vi "HexapodInitializeHardware.vi"(8 "error in (no error)":errorcluster, 11 "HexapodPI in":refnum<class "HexapodPI.lvclass">) -> (0 "error out":errorcluster, 2 "devaddress":string, 3 "HexapodPI out":refnum<class "HexapodPI.lvclass">)   [LabVIEW 2020, in "HexapodPI.lvclass"]
uses:
  HexapodPI.lvclass
  HexapodPI.lvclass/HexapodPI.ctl
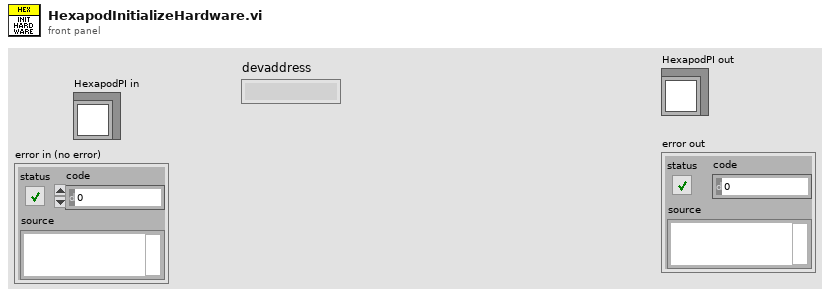
[diagram p1: front panel]
types:
  T1 = cluster{"connection ID":refnum<k5>, "VISA resource name out":refnum<visa-resource-name>, "connectiontype":enum16{"TCPIP", "Serial"}}
  T2 = cluster{"connection ID":refnum<k5>, "VISA resource name":refnum<visa-resource-name>, "Selector":enum16{"TCPIP", "Serial"}}
  T3 = cluster{"connection ID":refnum<k5>, "VISA Refnum out":refnum<visa-resource-name>, "Selector":enum16{"TCPIP", "Serial"}}
  T4 = cluster{"Strut 1 motion error":bool, "Strut 2 motion error":bool, "Strut 3 motion error":bool, "Strut 4 motion error":bool, "Strut 5 motion error":bool, "Strut 6 motion error":bool, "Axis A motion error":bool, "Axis B motion error":bool, "Strut 1 in motion":bool, "Strut 2 in motion":bool, "Strut 3 in motion":bool, "Strut 4 in motion":bool, "Strut 5 in motion":bool, "Strut 6 in motion":bool, "Axis A in motion":bool, "Axis B in motion":bool, "Hexapod is Initialized":bool, "Stage A is Initialized":bool, "Stage B is Initialized":bool, "Initialisation in progress":bool}
  T5 = typedef "PivotPoint_TypDef.ctl" = cluster{"R":cluster{"Value":dbl, "Min":dbl, "Max":dbl, "StepSize":dbl, "Tolerance":dbl, "ValueActual":dbl}, "S":cluster{"Value":dbl, "Min":dbl, "Max":dbl, "StepSize":dbl, "Tolerance":dbl, "ValueActual":dbl}, "T":cluster{"Value":dbl, "Min":dbl, "Max":dbl, "StepSize":dbl, "Tolerance":dbl, "ValueActual":dbl}}
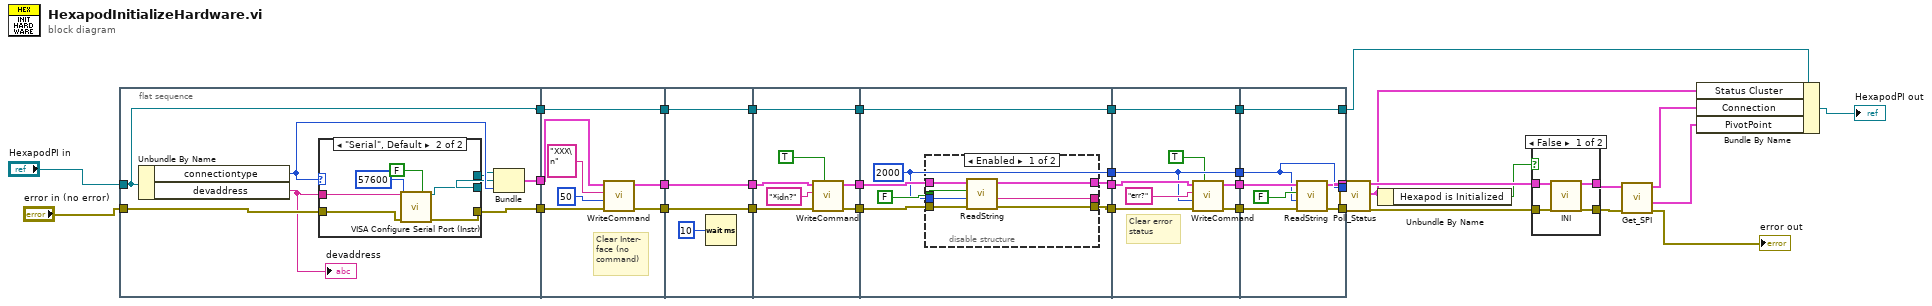
[diagram p0: block diagram]
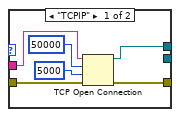
[diagram p3: hidden frame]
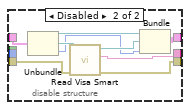
[diagram p4: hidden frame]
diagram:
  n1 = flat-sequence {
    tunnel: "error in (no error)" -> [w44]
    tunnel: [w43] -> w36
    tunnel: [w40] -> w35
    tunnel: "HexapodPI in" -> [w37]
    tunnel: [w37] -> w11
    tunnel: [w62] -> w34
    tunnel: [w60] -> w33
    tunnel: w36 -> [w61]
    tunnel: w35 -> [w58]
    tunnel: w11 -> [w57]
    tunnel: [w57] -> w8
    tunnel: w34 -> [w66]
    tunnel: [w66] -> w32
    tunnel: [w65] -> w31
    tunnel: w33 -> [w65]
    tunnel: [w64] -> w9
    tunnel: w8 -> [w64]
    tunnel: w32 -> [w74]
    tunnel: [w69] -> w30
    tunnel: w31 -> [w72]
    tunnel: [w71] -> w29
    tunnel: [w68] -> w10
    tunnel: w9 -> [w68]
    tunnel: w30 -> [w81]
    tunnel: [w76] -> w28
    tunnel: w29 -> [w79]
    tunnel: [w78] -> w27
    tunnel: [w77] -> w26
    tunnel: w10 -> [w75]
    tunnel: [w75] -> w6
    tunnel: w28 -> [w105]
    tunnel: [w104] -> w25
    tunnel: w27 -> [w101]
    tunnel: [w102] -> w24
    tunnel: w26 -> [w100]
    tunnel: [w100] -> w23
    tunnel: [w98] -> w7
    tunnel: w6 -> [w98]
    tunnel: w25 -> [w112]
    tunnel: [w111] -> w15
    tunnel: w24 -> [w109]
    tunnel: [w108] -> w14
    tunnel: w23 -> [w107]
    tunnel: [w107] -> w19
    tunnel: [w106] -> w5
    tunnel: w7 -> [w106]
    frame #0 {
      n2 = Unbundle By Name(w37) -> ("connectiontype"=w41:enum16{"TCPIP", "Serial"}, "devaddress"=w42:string)
      "devaddress" <- w42
      n3 = case shown="\"Serial\", Default" w41 {
        tunnel: w44 -> [w48 w52]
        tunnel: [w47 w55] -> w43
        tunnel: [w46 _] -> w38
        tunnel: w42 -> [w45 w53]
        tunnel: [_ w56] -> w39
        frame "TCPIP" {
          n4 = TCP Open Connection(address=w45, remote port or service name=u16 50000, timeout ms (60000)=5000, error in (no error)=w48) -> (connection ID=w46:refnum<k5>, error out=w47:errorcluster)  [unwired: 1 in]
        }
        frame "Serial", Default {
          n5 = call "VISA Configure Serial Port (Instr).vi"("VISA resource name"=w53, "Enable Termination\nChar (T)"=FALSE ("Enable Termination\nChar (T)"), "baud rate (9600)"=u32 57600, "error in (no error)"=w52) -> ("VISA resource name out"=w56:refnum<visa-resource-name>, "error out"=w55:errorcluster)  [unwired: 10 in]
        }
      }
      n6 = Bundle("connection ID"=w38, "VISA resource name out"=w39, "connectiontype"=w41) -> (w40:T1)  [unwired: 1 in]
    }
    frame #1 {
      # "Clear Inter-\nface (no\ncommand)"
      n7 = call "WriteCommand.vi"("error in (no error)"=w61, "timeout ms (0)"=50, "String"="XXX\n" ("Interface clear"), "Connection"=w58) -> ("error out"=w62:errorcluster, "Connection out"=w60:T2)  [unwired: 6 in]
    }
    frame #2 {
      n8 = Wait (ms)(milliseconds to wait=u32 10) -> ()  [unwired: 1 out]
    }
    frame #3 {
      n9 = call "WriteCommand.vi"("Attach Linefeed"=TRUE, "error in (no error)"=w74, "String"="*idn?" ("String to Send"), "Connection"=w72) -> ("error out"=w69:errorcluster, "Connection out"=w71:T2)  [unwired: 6 in]
    }
    frame #4 {
      w77 = 2000 ("timeout ms (0)")
      n10 = disable-structure shown="Enabled" {
        disable-tunnel: w81 -> [w88 w96]
        disable-tunnel: [w87 w89] -> _
        disable-tunnel: FALSE ("Strip spaces?") -> [w86 _]
        disable-tunnel: w79 -> [w85 w95]
        disable-tunnel: [w84 w92] -> w78
        disable-tunnel: w77 -> [w83 _]
        disable-tunnel: [w82 w97] -> w76
        frame Enabled {
          n11 = call "ReadString.vi"("error in (no error)"=w88, "timeout ms (0)"=w83, "Trim Spaces"=w86, "Connection"=w85) -> ("error out"=w82:errorcluster, "String out"=w87:string, "Connection out"=w84:T2)  [unwired: 5 in]
        }
        frame Disabled {
          n12 = Unbundle(w95) -> ("connection ID"=w93:refnum<k5>, "VISA resource name"=w94:refnum<visa-resource-name>, "Selector"=w90:enum16{"TCPIP", "Serial"})
          n13 = call "Read Visa Smart.vi"("error in (no error)"=w96, "VISA Refnum in"=w94) -> ("error out"=w97:errorcluster, "String"=w89:string, "VISA Refnum out"=w91:refnum<visa-resource-name>)  [unwired: 7 in]
          n14 = Bundle("connection ID"=w93, "VISA Refnum out"=w91, "Selector"=w90) -> (w92:T3)  [unwired: 1 in]
        }
      }
    }
    frame #5 {
      # "Clear error\nstatus"
      n15 = call "WriteCommand.vi"("Attach Linefeed"=TRUE, "error in (no error)"=w105, "timeout ms (0)"=w100, "String"="err?" ("String to Send"), "Connection"=w101) -> ("error out"=w104:errorcluster, "Connection out"=w102:T2)  [unwired: 5 in]
    }
    frame #6 {
      n16 = call "ReadString.vi"("error in (no error)"=w112, "timeout ms (0)"=w107, "Trim Spaces"=FALSE ("Strip spaces?"), "Connection"=w109) -> ("error out"=w111:errorcluster, "Connection out"=w108:T2)  [unwired: 5 in, 1 out]
    }
  }
  n17 = call "Poll_Status.vi"("Connection"=w14, "timeout ms (0)"=w19, "error in"=w15) -> ("Connection out"=w17:T2, "Status Cluster"=w4:T4, "error out"=w18:errorcluster)  [unwired: 14 in]
  n18 = Unbundle By Name(w4) -> ("Hexapod is Initialized"=w16:bool)
  n19 = case shown="False" w16 {
    tunnel: w17 -> [w116 w118]
    tunnel: [w115 w118] -> w20
    tunnel: w18 -> [w114 w117]
    tunnel: [w113 w117] -> w21
    frame False {
      n20 = call "INI.vi"("Connection"=w116, "error in"=w114) -> ("Connection out"=w115:T2, "error out"=w113:errorcluster)  [unwired: 16 in]
    }
    frame True {
    }
  }
  n21 = call "Get_SPI.vi"("error in (no error)"=w21, "Connection"=w20) -> ("error out"=→"error out":errorcluster, "PivotPoint"=w2:T5, "Connection out"=w3:T2)  [unwired: 6 in, 1 out]
  n22 = Bundle By Name(cluster=w5, "Status Cluster"=w4, "Connection"=w3, "PivotPoint"=w2) -> (→"HexapodPI out":refnum<class "HexapodPI.lvclass">)
